vi "AO_2Chan.vi"() -> ()   [LabVIEW 2021]
doc: "This example demonstrates how to generate a user-defined voltage using the analog output of a DAQ device."
uses:
  <vilib>/Utility/error.llb/DialogType.ctl
  <vilib>/DAQmx/write.llb/DAQmx Write (Analog 1D DBL NChan 1Samp).vi
  <vilib>/DAQmx/miscellaneous.llb/DAQmx Fill In Error Info.vi
  <vilib>/DAQmx/create/channels.llb/DAQmx Create Channel (AO-Voltage-Basic).vi
panel:
  in  "Control":enum16{"Up", "Zero", "Down"}[](array[ring])
  out "Output":dbl[](array[numeric])
  in  "Pulse Width":u32=100
  in  "Stop":bool
  in  "Max Voltage":dbl=10.0
  in  "Min Voltage":dbl=-10.0
  in  "Physical Channel(s)":tag="Dev2/ao0:1"
  # "Channel Settings"
  # "Output"
  # "The number of elements in the channel array\nmust equal the number of channels in the task."
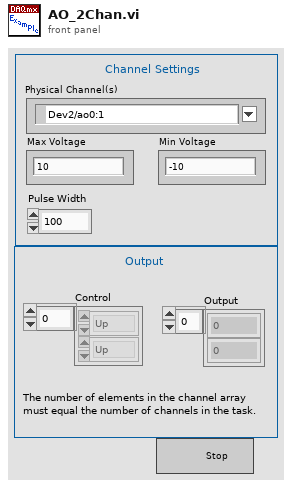
[diagram p1: front panel]
types:
  T1 = typedef "DialogType.ctl" = u16
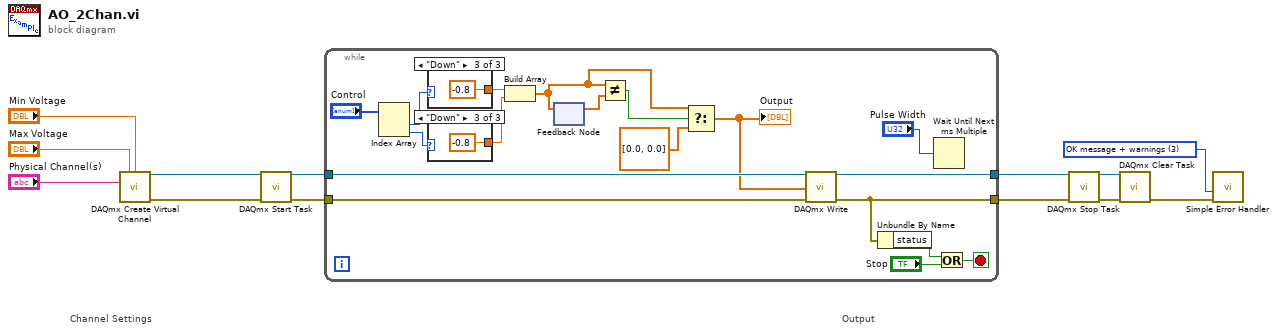
[diagram p0: block diagram]
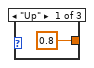
[diagram p2: hidden frame]
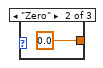
[diagram p3: hidden frame]
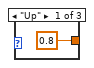
[diagram p4: hidden frame]
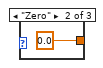
[diagram p5: hidden frame]
diagram:
  w1 = T1 3 items=["no dialog", "OK message", "continue or stop message", "OK message + warnings", "continue/stop + warnings"] ("type of dialog (OK msg:1)")
  # "Output"
  # "Channel Settings"
  n1 = call-poly <vilib>:"DAQmx Create Virtual Channel.vi"("maximum value"="Max Voltage", "minimum value"="Min Voltage", "physical channels"="Physical Channel(s)") -> ("task out"=w9:refnum<k21>, "error out"=w8:errorcluster)  [unwired: 11 in]
  n2 = call <vilib>:"DAQmx Start Task.vi"("task/channels in"=w9, "error in"=w8) -> ("task out"=w7:refnum<k21>, "error out"=w6:errorcluster)  [unwired: 12 in]
  n3 = while {
    tunnel: w7 -> [w31]
    tunnel: w6 -> [w30]
    tunnel: [w25] -> w4
    tunnel: [w29] -> w5
    stop <- w24 stop-if-true
    n4 = Index Array(array="Control") -> (element #1=w18:enum16{"Up", "Zero", "Down"}, element #2=w16:enum16{"Up", "Zero", "Down"})  [unwired: 2 in]
    n5 = case shown="\"Down\"" w18 {
      tunnel: [0.8 0.0 -0.8] -> w17
      frame "Up" {
      }
      frame "Zero" {
      }
      frame "Down" {
      }
    }
    n6 = case shown="\"Down\"" w16 {
      tunnel: [0.8 0.0 -0.8] -> w15
      frame "Up" {
      }
      frame "Zero" {
      }
      frame "Down" {
      }
    }
    n7 = Build Array(w17, w15) -> (w14:dbl[])
    n8 = feedback-in #1(w14) -> ()
    n9 = feedback #1() -> (w23:dbl[])  [unwired: 1 in]
    n10 = Not Equal?(x=w14, y=w23) -> (x != y?=w22:bool)
    n11 = Select(t=w14, s=w22, f=dbl[] [0.0, 0.0]) -> (s? t:f=w20:dbl[])
    "Output" <- w20
    n12 = call-poly <vilib>:"DAQmx Write.vi"("task/channels in"=w31, "data"=w20, "error in"=w30) -> ("task out"=w29:refnum<k21>, "error out"=w25:errorcluster)  [unwired: 10 in, 1 out]
    n13 = Unbundle By Name(w25) -> ("status"=w27:bool)
    n14 = Wait Until Next ms Multiple(millisecond multiple="Pulse Width") -> ()  [unwired: 1 out]
    n15 = Or(x=w27, y="Stop") -> (x .or. y?=w24:bool)
  }
  n16 = call <vilib>:"DAQmx Stop Task.vi"("task/channels in"=w5, "error in"=w4) -> ("task out"=w3:refnum<k21>, "error out"=w2:errorcluster)  [unwired: 12 in]
  n17 = call <vilib>:"DAQmx Clear Task.vi"("task in"=w3, "error in"=w2) -> ("error out"=w13:errorcluster)  [unwired: 13 in]
  n18 = call <vilib>:"Simple Error Handler.vi"("type of dialog (OK msg:1)"=w1, "error in (no error)"=w13) -> ()  [unwired: 3 in, 5 out]
